vi "lab4.vi"() -> ()   [LabVIEW 2021]
panel:
  out "Numeric":dbl
  out "8":bool
  out "7":bool
  out "1":bool
  out "3":bool
  out "6":bool
  out "5":bool
  out "4":bool
  out "?":bool
  out "?":bool
  out "?":bool
  out "?":bool
  out "?":bool
  out "?":bool
  out "?":bool
  in  "6":bool
  in  "7":bool
  in  "5":bool
  in  "4":bool
  in  "3":bool
  in  "2":bool
  in  "1":bool
  out "?":bool
  out "2":bool
  in  "0":bool
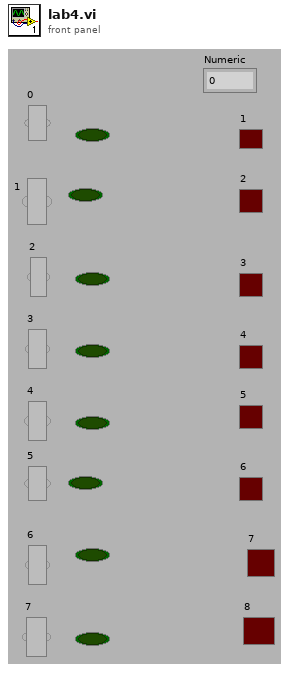
[diagram p1: front panel]
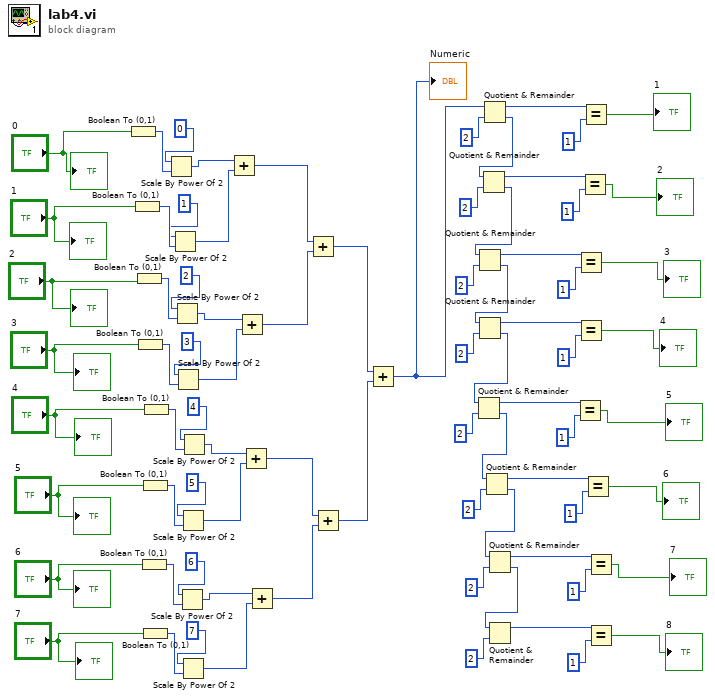
[diagram p0: block diagram]
diagram:
  n1 = Boolean To (0,1)(Boolean="0") -> (0, 1=w77:i16)
  n2 = Boolean To (0,1)(Boolean="1") -> (0, 1=w73:i16)
  n3 = Boolean To (0,1)(Boolean="2") -> (0, 1=w69:i16)
  n4 = Boolean To (0,1)(Boolean="3") -> (0, 1=w66:i16)
  n5 = Boolean To (0,1)(Boolean="6") -> (0, 1=w57:i16)
  n6 = Boolean To (0,1)(Boolean="5") -> (0, 1=w60:i16)
  n7 = Boolean To (0,1)(Boolean="7") -> (0, 1=w54:i16)
  n8 = Boolean To (0,1)(Boolean="4") -> (0, 1=w63:i16)
  n9 = Scale By Power Of 2(n=0, x=w77) -> (x*2^n=w75:i16)
  n10 = Scale By Power Of 2(n=1, x=w73) -> (x*2^n=w71:i16)
  n11 = Scale By Power Of 2(n=2, x=w69) -> (x*2^n=w52:i16)
  n12 = Scale By Power Of 2(n=3, x=w66) -> (x*2^n=w51:i16)
  n13 = Scale By Power Of 2(n=6, x=w57) -> (x*2^n=w48:i16)
  n14 = Scale By Power Of 2(n=5, x=w60) -> (x*2^n=w49:i16)
  n15 = Scale By Power Of 2(n=7, x=w54) -> (x*2^n=w47:i16)
  n16 = Scale By Power Of 2(n=4, x=w63) -> (x*2^n=w50:i16)
  n17 = Add(x=w75, y=w71) -> (x+y=w42:i16)
  n18 = Add(x=w52, y=w51) -> (x+y=w43:i16)
  n19 = Add(x=w50, y=w49) -> (x+y=w45:i16)
  n20 = Add(x=w48, y=w47) -> (x+y=w46:i16)
  n21 = Add(x=w42, y=w43) -> (x+y=w41:i16)
  n22 = Add(x=w45, y=w46) -> (x+y=w44:i16)
  n23 = Add(x=w41, y=w44) -> (x+y=w1:i16)
  "Numeric" <- w1
  n24 = Quotient & Remainder(x=w1, y=2) -> (x-y*floor(x/y)=w38:i32, floor(x/y)=w16:i32)
  n25 = Quotient & Remainder(x=w16, y=2) -> (x-y*floor(x/y)=w35:i32, floor(x/y)=w15:i32)
  n26 = Quotient & Remainder(x=w15, y=2) -> (x-y*floor(x/y)=w32:i32, floor(x/y)=w14:i32)
  n27 = Quotient & Remainder(x=w14, y=2) -> (x-y*floor(x/y)=w29:i32, floor(x/y)=w13:i32)
  n28 = Quotient & Remainder(x=w13, y=2) -> (x-y*floor(x/y)=w26:i32, floor(x/y)=w12:i32)
  n29 = Quotient & Remainder(x=w12, y=2) -> (x-y*floor(x/y)=w23:i32, floor(x/y)=w11:i32)
  n30 = Quotient & Remainder(x=w11, y=2) -> (x-y*floor(x/y)=w20:i32, floor(x/y)=w10:i32)
  n31 = Quotient & Remainder(x=w10, y=2) -> (x-y*floor(x/y)=w17:i32)  [unwired: 1 out]
  n32 = Equal?(x=w26, y=1) -> (x = y?=→"5":bool)
  n33 = Equal?(x=w32, y=1) -> (x = y?=→"3":bool)
  n34 = Equal?(x=w29, y=1) -> (x = y?=→"4":bool)
  n35 = Equal?(x=w35, y=1) -> (x = y?=→"2":bool)
  n36 = Equal?(x=w38, y=1) -> (x = y?=→"1":bool)
  n37 = Equal?(x=w23, y=1) -> (x = y?=→"6":bool)
  n38 = Equal?(x=w20, y=1) -> (x = y?=→"7":bool)
  n39 = Equal?(x=w17, y=1) -> (x = y?=→"8":bool)
  "?" <- "0"
  "?" <- "3"
  "?" <- "1"
  "?" <- "2"
  "?" <- "5"
  "?" <- "4"
  "?" <- "7"
  "?" <- "6"
